vi "Show Battery Current.vi"(8 "error in (no error)":errorcluster) -> (0 "error out":errorcluster)   [LabVIEW 2015]
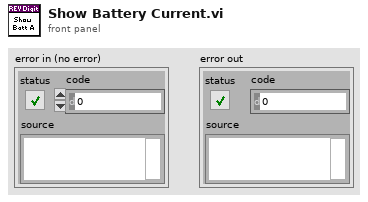
[diagram p1: front panel]
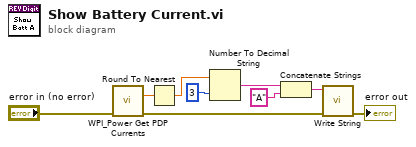
[diagram p0: block diagram]
diagram:
  n1 = call <vilib>:"WPI_Power Get PDP Currents.vi"("error in"="error in (no error)") -> ("current (A)"=w8:dbl, "error out"=w7:errorcluster)  [unwired: 12 in, 1 out]
  n2 = Round To Nearest(number=w8) -> (nearest integer value=w6:dbl)
  n3 = Number To Decimal String(number=w6, width (-)=i16 3) -> (decimal integer string=w4:string)
  n4 = Concatenate Strings(w4, "A" ("string")) -> (w2:string)
  n5 = call "Write String.vi"("error in (no error)"=w7, "String"=w2) -> ("error out"=→"error out":errorcluster)  [unwired: 9 in]
